vi "Read Coordinates.CAD Cluster.vi"(8 "error in (no error)":errorcluster, 11 "CAD Dispense in":refnum<class "CAD Dispense.lvclass">) -> (0 "error out":errorcluster, 2 "Coordinates.CAD Cluster":T1(array[cluster]), 3 "CAD Dispense out":refnum<class "CAD Dispense.lvclass">)   [LabVIEW 2016, in "CAD Dispense.lvclass"]
uses:
  CAD Dispense.lvclass
  CAD Dispense.lvclass/CAD Dispense.ctl
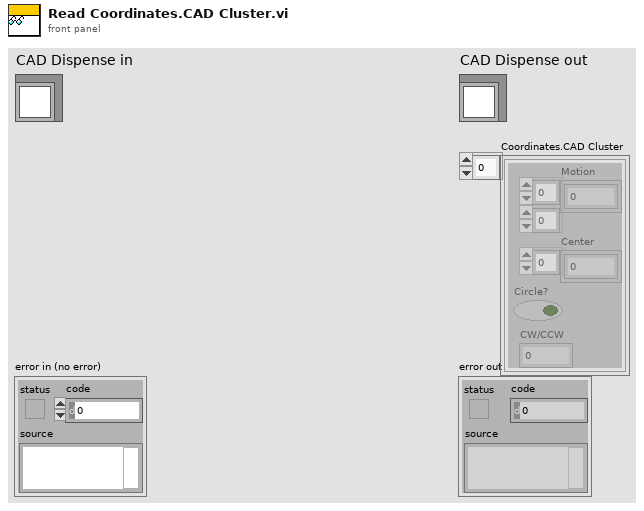
[diagram p1: front panel]
types:
  T1 = cluster{"Motion":dbl[][], "Center":dbl[], "Circle?":bool, "CW/CCW":dbl}[]
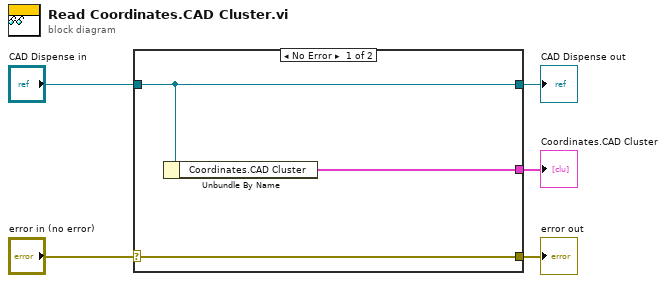
[diagram p0: block diagram]
diagram:
  n1 = case shown="No Error" "error in (no error)" {
    selector: "error in (no error)" -> [w8 w9]
    tunnel: [w8 w9] -> w4
    tunnel: [w7 w10] -> w2
    tunnel: "CAD Dispense in" -> [w7 w10]
    tunnel: [w6 _] -> w1
    frame No Error {
      n2 = Unbundle By Name(w7) -> ("Coordinates.CAD Cluster"=w6:T1)
    }
    frame Error {
    }
  }
  "error out" <- w4
  "CAD Dispense out" <- w2
  "Coordinates.CAD Cluster" <- w1
